vi "GetLastTileInRiver.vi"() -> ()   [LabVIEW 2025]
uses:
  Controls/Player.ctl
panel:
  out "LastTile":u16(ring)
  in  "Player":T1
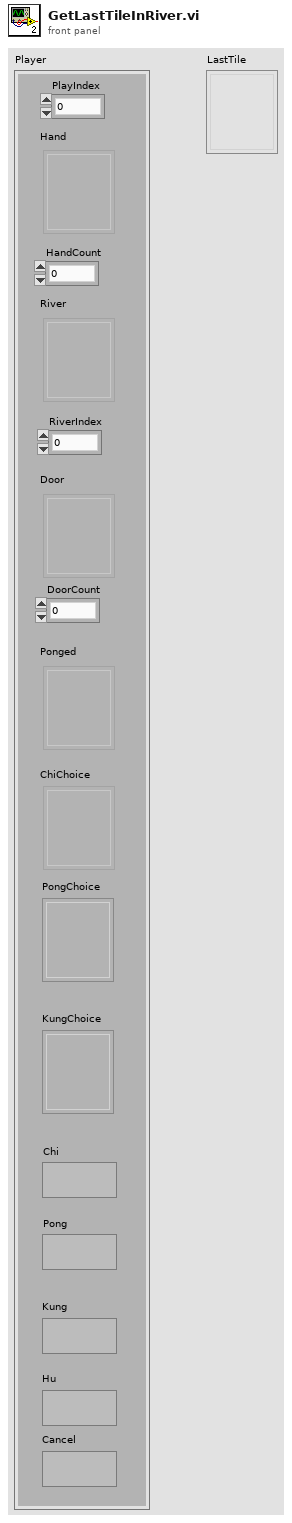
[diagram p1: front panel]
types:
  T1 = typedef "Player.ctl" = cluster{"PlayIndex":u16, "Hand":u16[], "HandCount":u16, "RiverIndex":u16, "Door":u16[], "DoorCount":u16, "Ponged":u16[], "ChiChoice":u16[][], "River":u16[][], "Chi":bool, "Pong":bool, "Kung":bool, "Hu":bool, "Cancel":bool, "PongChoice":u16, "KungChoice":u16}
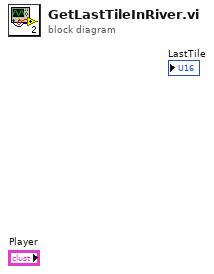
[diagram p0: block diagram]
diagram:
